vi "DAQ Loop.vi"(8 "error in (no error)":errorcluster, 10 "Reference Cluster":T1, 11 "DAQ Queue":refnum<queue>) -> (0 "error out":errorcluster, 3 "Stop":bool)   [LabVIEW 2017]
doc: "This VI is used to control and communicate with the DAQ cards.\n\nTo make it efficient, I also used this VI to control the graphs of the Main FP through the reference cluster."
uses:
  DAQ States.ctl
  <vilib>/DAQmx/write.llb/DAQmx Write (Analog Wfm 1Chan NSamp).vi
  <vilib>/DAQmx/write.llb/DAQmx Write (Digital Bool 1Line 1Point).vi
  <vilib>/DAQmx/write.llb/DAQmx Write (Analog 1D DBL 1Chan NSamp).vi
  <vilib>/DAQmx/read.llb/DAQmx Read (Counter 1D DBL 1Chan NSamp).vi
  <vilib>/Analysis/baseanly.llb/Mean (DBL).vi
  <vilib>/DAQmx/configure/timing.llb/DAQmx Timing (Sample Clock).vi
  <vilib>/DAQmx/miscellaneous.llb/DAQmx Fill In Error Info.vi
  <resource>/objmgr/daqmx.rc
  <vilib>/Analysis/NI_AALBase.lvlib
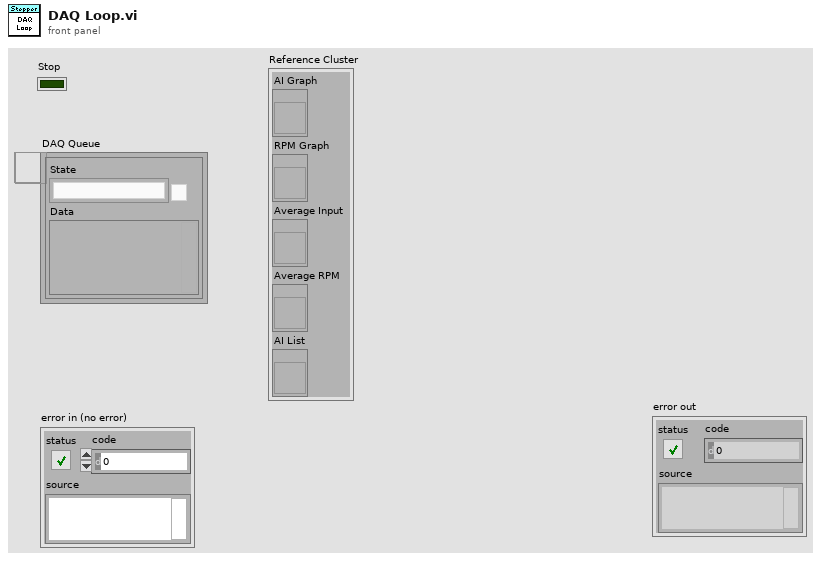
[diagram p1: front panel]
types:
  T1 = cluster{"AI Graph":refnum<vi>, "RPM Graph":refnum<vi>, "Average Input":refnum<vi>, "Average RPM":refnum<vi>, "AI List":refnum<vi>}
  T2 = cluster{"Torque Percentage":sgl, "Enable Drive":bool}
  T3 = typedef "DAQ States.ctl" = enum16{"Init", "Exit", "Update Settings", "Pause", "Update Square", "Update Duration"}
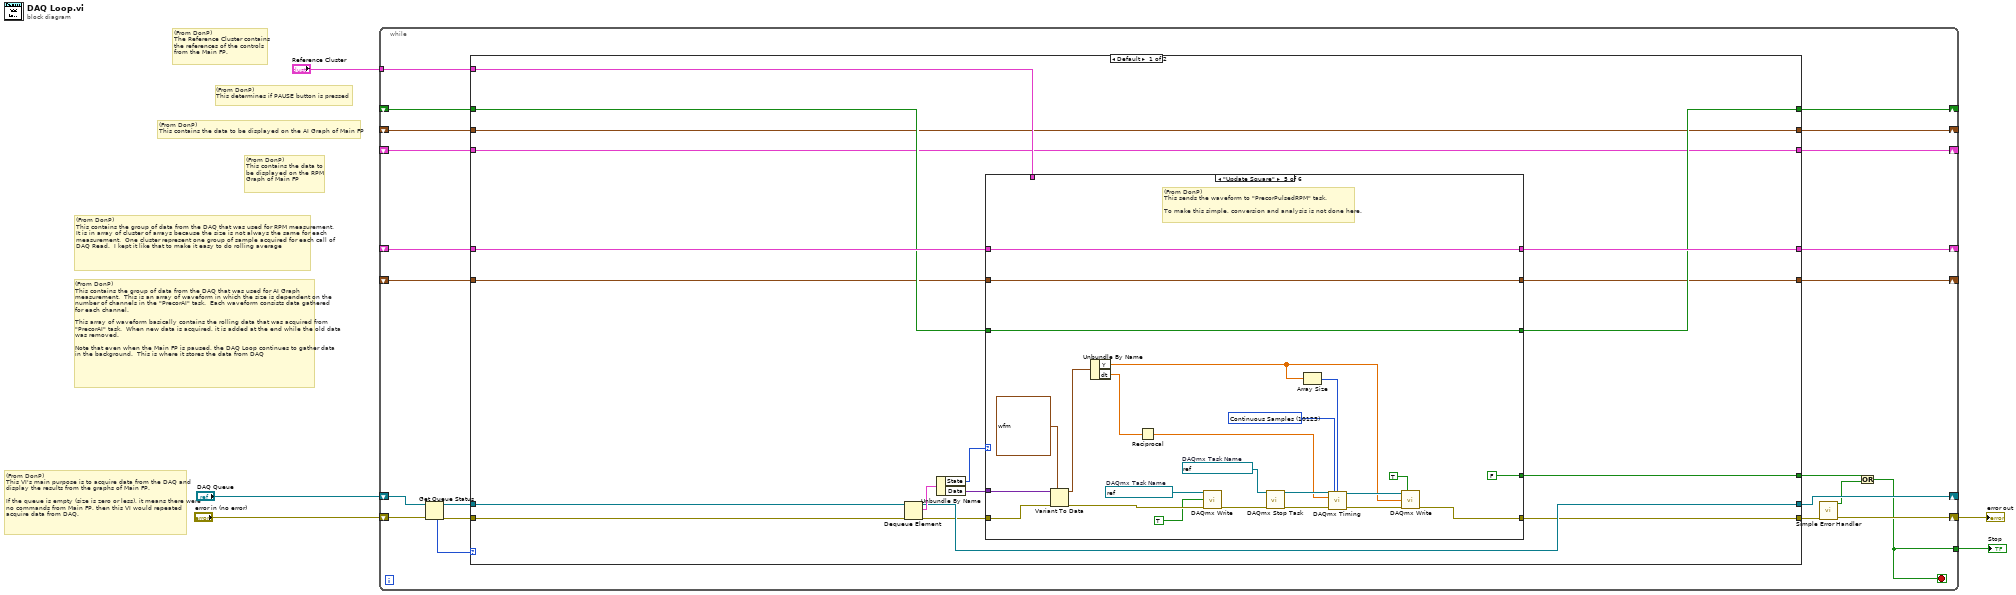
[diagram p0: block diagram]
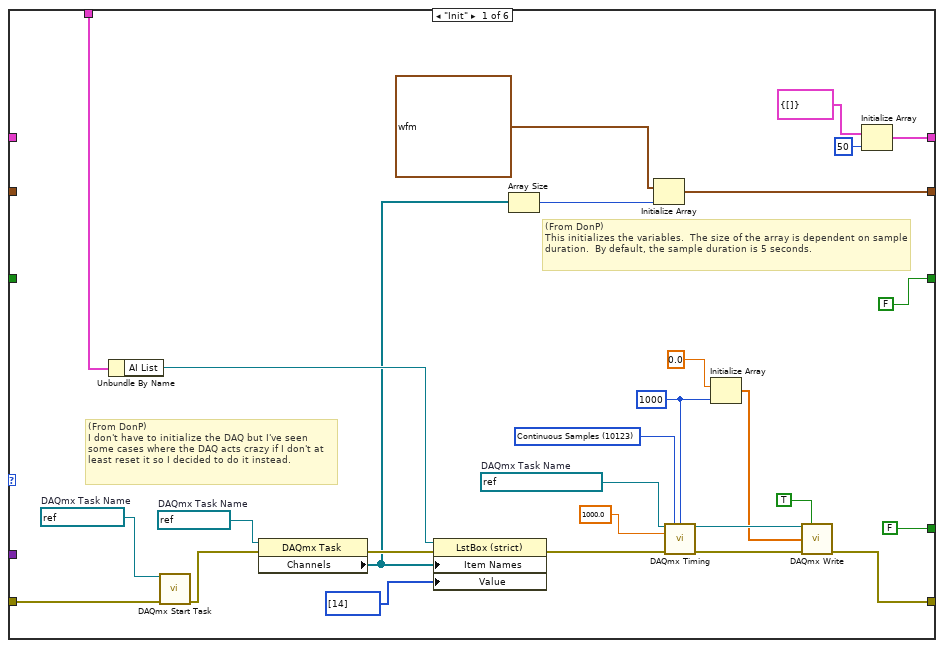
[diagram p2: hidden frame]
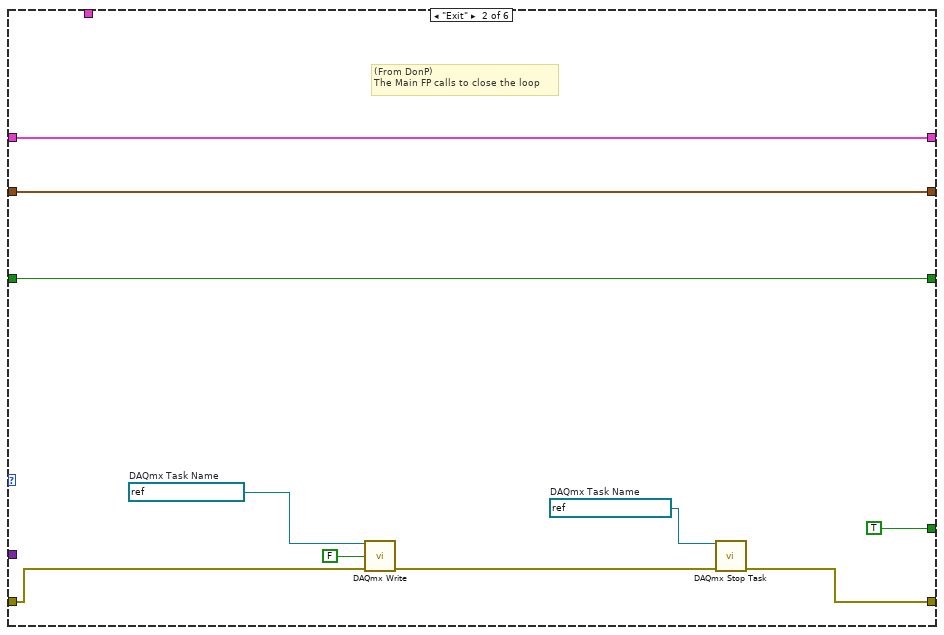
[diagram p3: hidden frame]
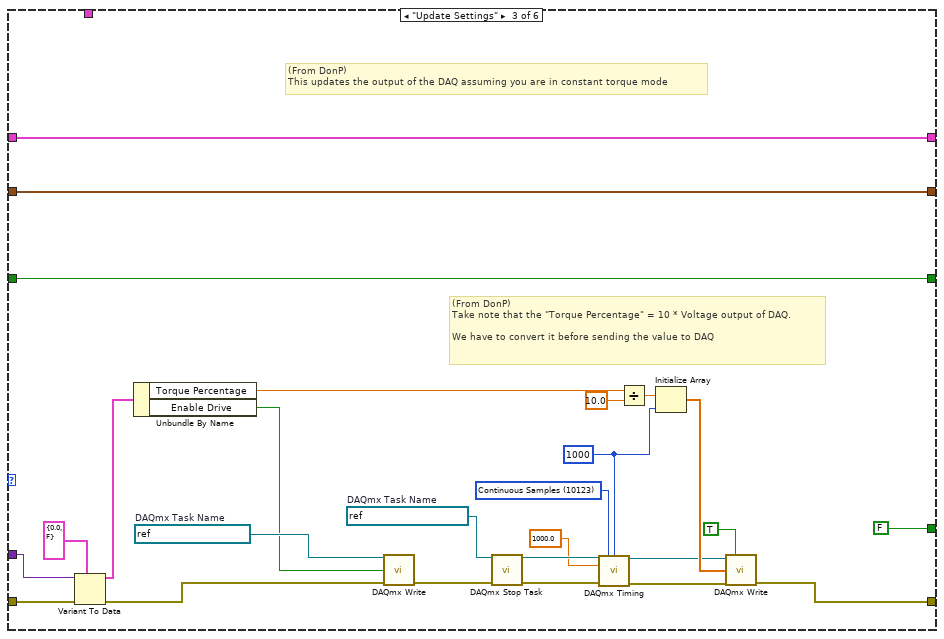
[diagram p4: hidden frame]
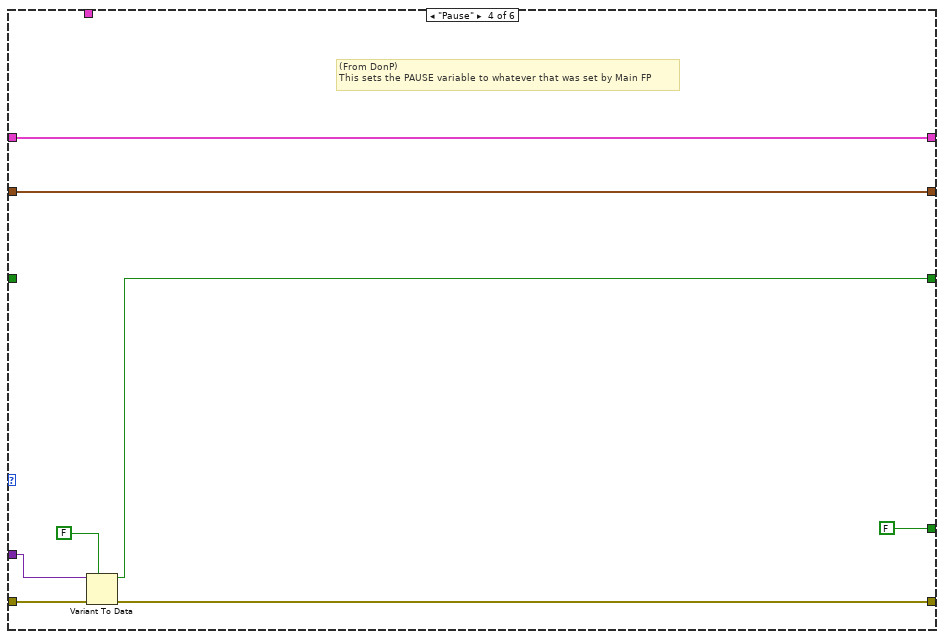
[diagram p5: hidden frame]
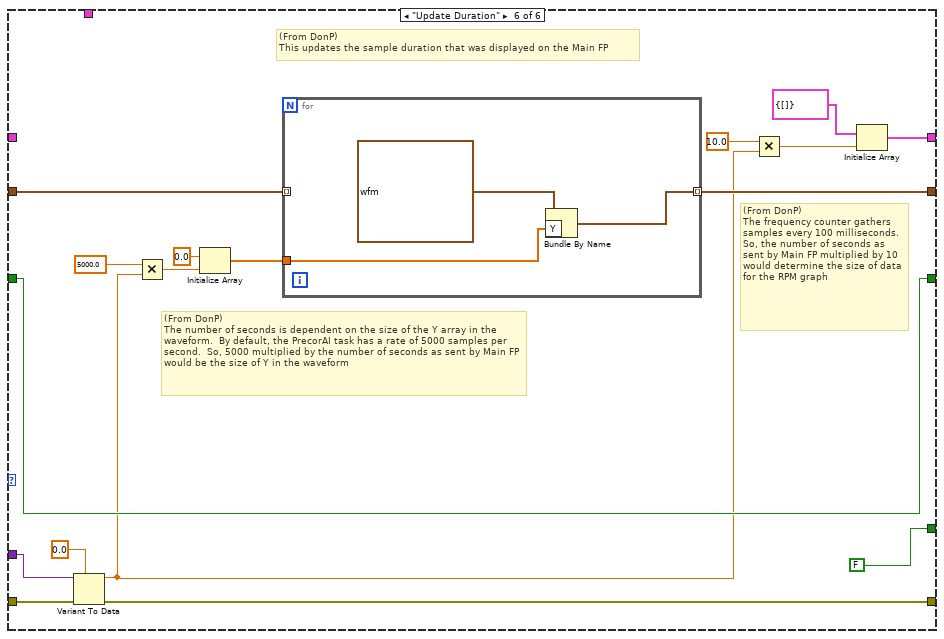
[diagram p6: hidden frame]
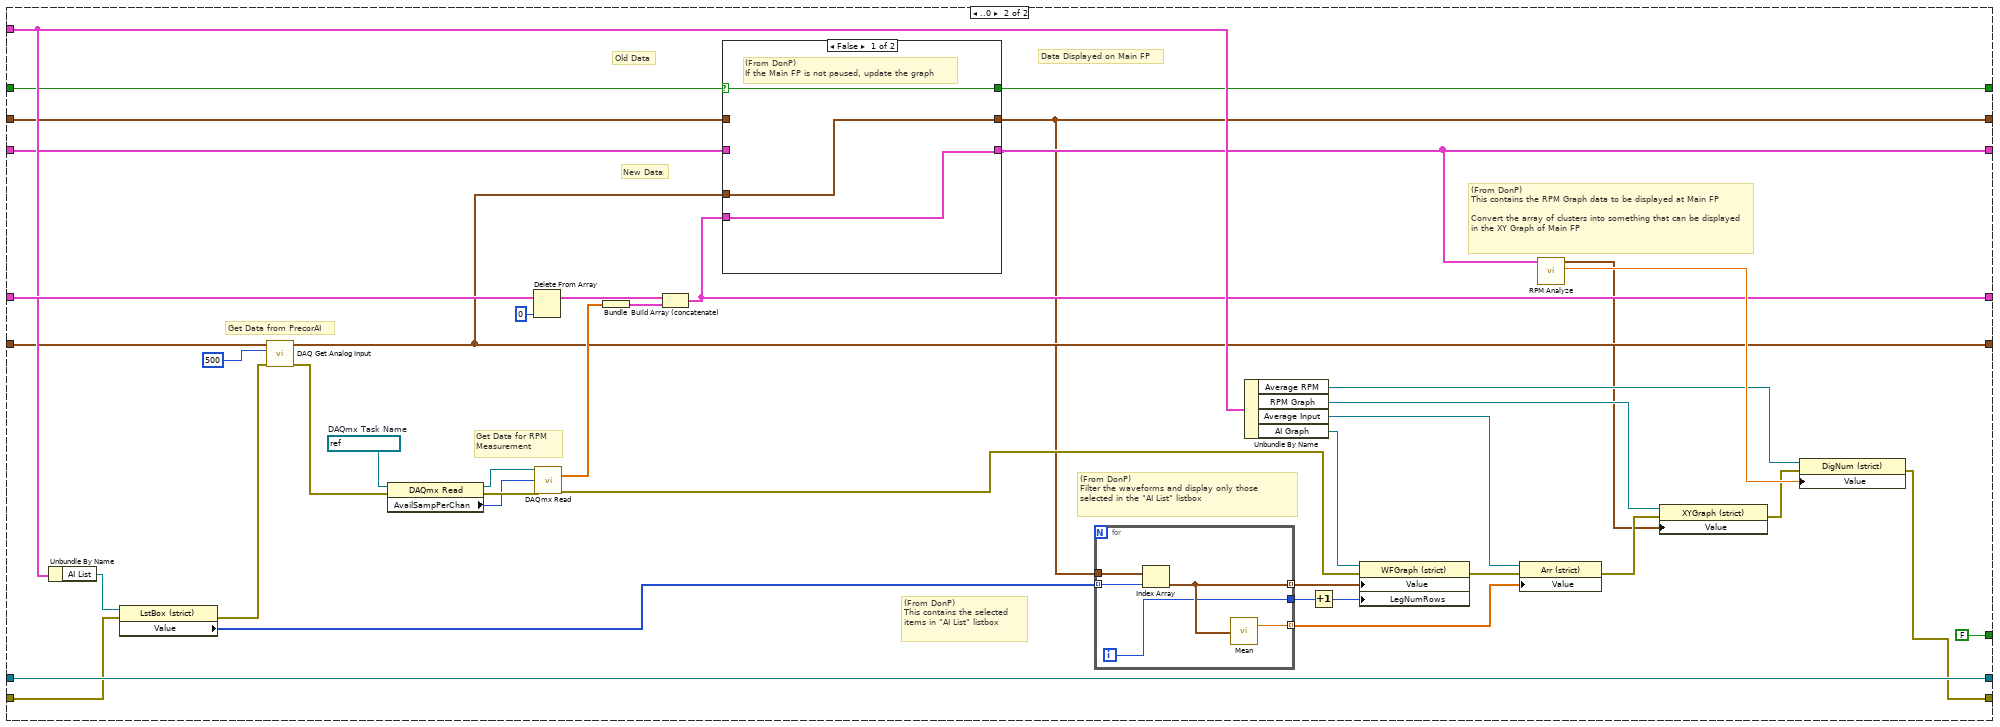
[diagram p7: hidden frame]
diagram:
  # "(From DonP)\nThis contains the group of data from the DAQ that was used for AI Graph measurement.  This is an array of waveform in which the size is dependent on the number of channels in the \"PrecorAI\" task.  Each waveform consists data gathered for each channel.\n\nThis array of waveform basically contains the rolling data that was acquired from \"PrecorAI\" task.  When new data is acquired, it is added at the end while the old data was removed.\n\nNote that even when the Main FP is paused, the DAQ Loop continues to gather data in the background.  This is where it stores the data from DAQ"
  # "(From DonP)\nThis contains the group of data from the DAQ that was used for RPM measurement.  It is in array of cluster of arrays because the size is not always the same for each measurement.  One cluster represent one group of sample acquired for each call of DAQ Read.  I kept it like that to make it easy to do rolling average"
  # "(From DonP)\nThis contains the data to be displayed on the RPM Graph of Main FP"
  # "(From DonP)\nThis contains the data to be displayed on the AI Graph of Main FP"
  # "(From DonP)\nThis determines if PAUSE button is pressed"
  # "(From DonP)\nThe Reference Cluster contains the references of the controls from the Main FP."
  # "(From DonP)\nThis VI's main purpose is to acquire data from the DAQ and display the results from the graphs of Main FP.\n\nIf the queue is empty (size is zero or less), it means there were no commands from Main FP, then this VI would repeated acquire data from DAQ."
  n1 = while {
    shift-right: [w21] -> w4
    shift-left: "error in (no error)" -> [w27]
    shift-right: [w22] -> _
    shift-left: "DAQ Queue" -> [w26]
    tunnel: [w10] -> w3
    tunnel: "Reference Cluster" -> [w19]
    shift-right: [w18] -> _
    shift-left: _ -> [w17]
    shift-right: [w16] -> _
    shift-left: _ -> [w15]
    shift-right: [w14] -> _
    shift-left: _ -> [w13]
    shift-right: [w9] -> _
    shift-left: _ -> [w7]
    shift-right: [w8] -> _
    shift-left: _ -> [w6]
    stop <- w10 stop-if-true
    n2 = Get Queue Status(queue=w26, error in (no error)=w27) -> (queue out=w25:refnum<queue>, error out=w24:errorcluster, # elements in queue=w23:i32)  [unwired: 1 in, 5 out]
    n3 = case shown="Default" w23 {
      tunnel: w25 -> [w45 w203]
      tunnel: w24 -> [w44 w185]
      tunnel: [w42 w203] -> w22
      tunnel: [w38 w191] -> w20
      tunnel: [w37 FALSE] -> w12
      tunnel: w19 -> [w32 w190]
      tunnel: [w36 w173] -> w18
      tunnel: w17 -> [w35 w196]
      tunnel: [w34 w174] -> w16
      tunnel: w15 -> [w33 w175]
      tunnel: [w31 w169] -> w14
      tunnel: w13 -> [w30 w186]
      tunnel: [w29 w165] -> w9
      tunnel: [w28 w166] -> w8
      tunnel: w7 -> [w29 w168]
      tunnel: w6 -> [w28 w167]
      frame Default {
        n4 = Dequeue Element(queue=w45, error in (no error)=w44) -> (queue out=w42:refnum<queue>, element=w43:cluster{"State":T3, "Data":variant}, error out=w39:errorcluster)  [unwired: 1 in, 1 out]
        n5 = Unbundle By Name(w43) -> ("State"=w41:T3, "Data"=w40:variant)
        n6 = case shown="\"Update Square\"" w41 {
          tunnel: w40 -> [_ _ w108 w115 w140 w155]
          tunnel: w39 -> [w71 w81 w107 w114 w139 w156]
          tunnel: [w56 w74 w98 w112 w135 w153] -> w38
          tunnel: [FALSE TRUE FALSE FALSE FALSE FALSE] -> w37
          tunnel: [w68 w79 w101 w116 w136 w151] -> w36
          tunnel: w35 -> [_ w79 w101 w116 w136 _]
          tunnel: [FALSE w78 w97 w111 w134 w158] -> w34
          tunnel: w33 -> [_ w78 w97 _ w134 w158]
          tunnel: w32 -> [w66 _ _ _ _ _]
          tunnel: [w58 w77 w96 w110 w133 w147] -> w31
          tunnel: w30 -> [_ w77 w96 w110 w133 w148]
          frame "Init" {
            w49 = 1000 ("samples per channel")
            w50 = 10123 items=["Finite Samples"=10178, "Continuous Samples"=10123, "Hardware Timed Single Point"=12522] ("sample mode")
            w51 = refnum<k21> "PrecorPulsedRPM"  # DAQmx Task Name
            w65 = refnum<k21> "PrecorAI"  # DAQmx Task Name
            w72 = refnum<k21> "PrecorCTR"  # DAQmx Task Name
            # "(From DonP)\nI don't have to initialize the DAQ but I've seen some cases where the DAQ acts crazy if I don't at least reset it so I decided to do it instead."
            # "(From DonP)\nThis initializes the variables.  The size of the array is dependent on sample duration.  By default, the sample duration is 5 seconds."
            n7 = Unbundle By Name(w66) -> ("AI List"=w63:refnum<vi>)
            n8 = call <vilib>:"DAQmx Start Task.vi"("task/channels in"=w72, "error in"=w71) -> ("error out"=w64:errorcluster)  [unwired: 12 in, 1 out]
            n9 = property class="DAQmx Task"(reference=w65, error in=w64) -> (error out=w62:errorcluster, "Channels"=w59:refnum<k21>[])  [unwired: 1 out]
            n10 = property class="LstBox (strict)"(reference=w63, error in=w62, "Item Names"=w59, "Value"=i32[] [14]) -> (error out=w52:errorcluster)  [unwired: 1 out]
            n11 = Array Size(array=w59) -> (size(s)=w60:i32)
            n12 = Initialize Array(waveform(dbl) {"t0"=timestamp(0 s since 1904-01-01), "dt"=0.0002, "Y"=array[25001 elements]} ("Waveform"), w60) -> (w58:waveform(dbl)[])
            n13 = call-poly <vilib>:"DAQmx Timing.vi"("task/channels in"=w51, "sample mode"=w50, "samples per channel"=w49, "rate"=1000.0, "error in"=w52) -> ("task out"=w54:refnum<k21>, "error out"=w53:errorcluster)  [unwired: 9 in]
            n14 = Initialize Array(0.0, w49) -> (w47:dbl[])
            n15 = call-poly <vilib>:"DAQmx Write.vi"("task/channels in"=w54, "auto start"=TRUE, "data"=w47, "error in"=w53) -> ("error out"=w56:errorcluster)  [unwired: 9 in, 2 out]
            n16 = Initialize Array(cluster{dbl[]} {[]}, 50 ("dimension size")) -> (w68:cluster{dbl[]}[])
          }
          frame "Exit" {
            w76 = refnum<k21> "PrecorPulsedRPM"  # DAQmx Task Name
            w82 = refnum<k21> "PrecorMCEnable"  # DAQmx Task Name
            # "(From DonP)\nThe Main FP calls to close the loop"
            n17 = call-poly <vilib>:"DAQmx Write.vi"("task/channels in"=w82, "data"=FALSE, "error in"=w81) -> ("error out"=w75:errorcluster)  [unwired: 10 in, 2 out]
            n18 = call <vilib>:"DAQmx Stop Task.vi"("task/channels in"=w76, "error in"=w75) -> ("error out"=w74:errorcluster)  [unwired: 12 in, 1 out]
          }
          frame "Update Settings" {
            w84 = 1000 ("samples per channel")
            w85 = 10123 items=["Finite Samples"=10178, "Continuous Samples"=10123, "Hardware Timed Single Point"=12522] ("sample mode")
            w92 = refnum<k21> "PrecorPulsedRPM"  # DAQmx Task Name
            w104 = refnum<k21> "PrecorMCEnable"  # DAQmx Task Name
            # "(From DonP)\nTake note that the \"Torque Percentage\" = 10 * Voltage output of DAQ.\n\nWe have to convert it before sending the value to DAQ"
            # "(From DonP)\nThis updates the output of the DAQ assuming you are in constant torque mode"
            n19 = Variant To Data(error in=w107, type=T2 {"Torque Percentage"=0.0, "Enable Drive"=FALSE} ("Target Settings"), Variant=w108) -> (data=w105:T2, error out=w102:errorcluster)
            n20 = Unbundle By Name(w105) -> ("Torque Percentage"=w100:sgl, "Enable Drive"=w103:bool)
            n21 = call-poly <vilib>:"DAQmx Write.vi"("task/channels in"=w104, "data"=w103, "error in"=w102) -> ("error out"=w93:errorcluster)  [unwired: 10 in, 2 out]
            n22 = call <vilib>:"DAQmx Stop Task.vi"("task/channels in"=w92, "error in"=w93) -> ("task out"=w90:refnum<k21>, "error out"=w87:errorcluster)  [unwired: 12 in]
            n23 = call-poly <vilib>:"DAQmx Timing.vi"("task/channels in"=w90, "sample mode"=w85, "samples per channel"=w84, "rate"=1000.0, "error in"=w87) -> ("task out"=w89:refnum<k21>, "error out"=w88:errorcluster)  [unwired: 9 in]
            n24 = Divide(x=w100, y=sgl 10.0) -> (x/y=w95:sgl)
            n25 = Initialize Array(w95, w84) -> (w94:sgl[])
            n26 = call-poly <vilib>:"DAQmx Write.vi"("task/channels in"=w89, "auto start"=TRUE, "data"=w94, "error in"=w88) -> ("error out"=w98:errorcluster)  [unwired: 9 in, 2 out]
          }
          frame "Pause" {
            # "(From DonP)\nThis sets the PAUSE variable to whatever that was set by Main FP"
            n27 = Variant To Data(error in=w114, type=FALSE, Variant=w115) -> (data=w111:bool, error out=w112:errorcluster)
          }
          frame "Update Square" {
            w125 = 10123 items=["Finite Samples"=10178, "Continuous Samples"=10123, "Hardware Timed Single Point"=12522] ("sample mode")
            w131 = refnum<k21> "PrecorPulsedRPM"  # DAQmx Task Name
            w138 = refnum<k21> "PrecorMCEnable"  # DAQmx Task Name
            # "(From DonP)\nThis sends the waveform to \"PrecorPulsedRPM\" task.\n\nTo make this simple, conversion and analysis is not done here."
            n28 = Variant To Data(error in=w139, type=waveform(dbl) {"t0"=timestamp(0 s since 1904-01-01), "dt"=1.0, "Y"=[]} ("Waveform"), Variant=w140) -> (data=w122:waveform(dbl), error out=w137:errorcluster)
            n29 = Unbundle By Name(w122) -> ("Y"=w120:dbl[], "dt"=w119:dbl)
            n30 = Reciprocal(x=w119) -> (1/x=w118:dbl)
            n31 = call-poly <vilib>:"DAQmx Write.vi"("task/channels in"=w138, "data"=TRUE, "error in"=w137) -> ("error out"=w132:errorcluster)  [unwired: 10 in, 2 out]
            n32 = call <vilib>:"DAQmx Stop Task.vi"("task/channels in"=w131, "error in"=w132) -> ("task out"=w129:refnum<k21>, "error out"=w126:errorcluster)  [unwired: 12 in]
            n33 = Array Size(array=w120) -> (size(s)=w121:i32)
            n34 = call-poly <vilib>:"DAQmx Timing.vi"("task/channels in"=w129, "sample mode"=w125, "samples per channel"=w121, "rate"=w118, "error in"=w126) -> ("task out"=w128:refnum<k21>, "error out"=w127:errorcluster)  [unwired: 9 in]
            n35 = call-poly <vilib>:"DAQmx Write.vi"("task/channels in"=w128, "auto start"=TRUE, "data"=w120, "error in"=w127) -> ("error out"=w135:errorcluster)  [unwired: 9 in, 2 out]
          }
          frame "Update Duration" {
            # "(From DonP)\nThe frequency counter gathers samples every 100 milliseconds.  So, the number of seconds as sent by Main FP multiplied by 10 would determine the size of data for the RPM graph"
            # "(From DonP)\nThe number of seconds is dependent on the size of the Y array in the waveform.  By default, the PrecorAI task has a rate of 5000 samples per second.  So, 5000 multiplied by the number of seconds as sent by Main FP would be the size of Y in the waveform"
            # "(From DonP)\nThis updates the sample duration that was displayed on the Main FP"
            n36 = Variant To Data(error in=w156, type=0.0, Variant=w155) -> (data=w146:dbl, error out=w153:errorcluster)
            n37 = Multiply(x=5000.0, y=w146) -> (x*y=w144:dbl)
            n38 = Initialize Array(0.0 ("element"), w144) -> (w142:dbl[])
            n39 = for {
              tunnel: w148 -> [_] mode=indexing
              tunnel: [w160] -> w147 mode=indexing
              tunnel: w142 -> [w159]
              n40 = Bundle By Name(cluster=waveform(dbl) {"t0"=timestamp(0 s since 1904-01-01), "dt"=0.0002, "Y"=[]} ("Waveform"), "Y"=w159) -> (w160:waveform(dbl))
            }
            n41 = Multiply(x=10.0, y=w146) -> (x*y=w150:dbl)
            n42 = Initialize Array(cluster{dbl[]} {[]}, w150) -> (w151:cluster{dbl[]}[])
          }
        }
      }
      frame ..0 {
        w201 = refnum<k21> "PrecorCTR"  # DAQmx Task Name
        # "(From DonP)\nThis contains the RPM Graph data to be displayed at Main FP\n\nConvert the array of clusters into something that can be displayed in the XY Graph of Main FP"
        # "(From DonP)\nThis contains the selected items in \"AI List\" listbox"
        # "(From DonP)\nFilter the waveforms and display only those selected in the \"AI List\" listbox"
        # "Get Data for RPM Measurement"
        # "Get Data from PrecorAI"
        # "Data Displayed on Main FP"
        # "New Data"
        # "Old Data"
        n43 = Unbundle By Name(w190) -> ("AI List"=w188:refnum<vi>)
        n44 = property class="LstBox (strict)"(reference=w188, error in=w185) -> (error out=w184:errorcluster, "Value"=w172:i32[])  [unwired: 1 out]
        n45 = call "DAQ Get Analog Input.vi"("error in (no error)"=w184, "Samples"=500 ("number of samples per channel"), "Waveforms In"=w186) -> ("error out"=w183:errorcluster, "Waveforms Out"=w169:waveform(dbl)[])  [unwired: 7 in]
        n46 = property class="DAQmx Read"(reference=w201, error in=w183) -> (reference out=w200:refnum<k21>, error out=w199:errorcluster, "AvailSampPerChan"=w198:u32)
        n47 = Delete From Array(array=w196, index=0) -> (array with subset deleted=w195:cluster{"data":dbl[]}[])  [unwired: 1 in, 1 out]
        n48 = call-poly <vilib>:"DAQmx Read.vi"("task/channels in"=w200, "number of samples per channel"=w198, "error in"=w199) -> ("data"=w194:dbl[], "error out"=w189:errorcluster)  [unwired: 10 in, 1 out]
        n49 = Bundle("data"=w194) -> (w193:cluster{"data":dbl[]})  [unwired: 1 in]
        n50 = Build Array (concatenate)(w195, w193) -> (w173:cluster{"data":dbl[]}[])
        n51 = case shown="False" w175 {
          selector: w175 -> [w211 w214]
          tunnel: [w211 w214] -> w174
          tunnel: w173 -> [w209 _]
          tunnel: w169 -> [w210 _]
          tunnel: [w210 w213] -> w165
          tunnel: [w209 w212] -> w166
          tunnel: w168 -> [_ w213]
          tunnel: w167 -> [_ w212]
          frame False {
            # "(From DonP)\nIf the Main FP is not paused, update the graph"
          }
          frame True {
            # "(From DonP)\nIf the Main FP is paused, do not update the graph"
          }
        }
        n52 = for {
          tunnel: w165 -> [w208]
          tunnel: w172 -> [w207] mode=indexing
          tunnel: [w205] -> w171 mode=indexing
          tunnel: [w206] -> w170 mode=indexing
          tunnel: [w204] -> w163
          i -> [w204]
          n53 = Index Array(array=w208, index=w207) -> (element=w205:waveform(dbl))
          n54 = call-poly <vilib>:"Mean.vi"("X"=w205) -> ("mean"=w206:dbl)  [unwired: 1 out]
        }
        n55 = Unbundle By Name(w190) -> ("Average RPM"=w177:refnum<vi>, "RPM Graph"=w179:refnum<vi>, "Average Input"=w181:refnum<vi>, "AI Graph"=w182:refnum<vi>)
        n56 = Increment(x=w163) -> (x+1=w162:i32)
        n57 = property class="WFGraph (strict)"(reference=w182, error in=w189, "Value"=w171, "LegNumRows"=w162) -> (error out=w180:errorcluster)  [unwired: 1 out]
        n58 = property class="Arr (strict)"(reference=w181, error in=w180, "Value"=w170) -> (error out=w178:errorcluster)  [unwired: 1 out]
        n59 = call "RPM Analyze.vi"("RPM Data"=w166) -> ("Mean RPM"=w192:dbl, "Output XY Graph"=w164:cluster{"X":dbl, "Y":dbl}[])  [unwired: 9 in]
        n60 = property class="XYGraph (strict)"(reference=w179, error in=w178, "Value"=w164) -> (error out=w176:errorcluster)  [unwired: 1 out]
        n61 = property class="DigNum (strict)"(reference=w177, error in=w176, "Value"=w192) -> (error out=w191:errorcluster)  [unwired: 1 out]
      }
    }
    n62 = call <vilib>:"Simple Error Handler.vi"("error in (no error)"=w20) -> ("error?"=w11:bool, "error out"=w21:errorcluster)  [unwired: 4 in, 3 out]
    n63 = Or(x=w12, y=w11) -> (x .or. y?=w10:bool)
  }
  "Stop" <- w3
  "error out" <- w4
